vi "Configure Alarm Delay Math.vi"(0 "VISA resource name":refnum<visa-resource-name>, 5 "Math Channel (001)":string="001", 7 "Alarm Delay Time":cluster{"Hour":i32, "Min":i32, "Sec":i32}={"Hour"=0, "Min"=0, "Sec"=10} {"Sec" min=0 max=59; "Min" min=0 max=59; "Hour" min=0 max=24}, 11 "error in (no error)":errorcluster) -> (4 "VISA resource name out":refnum<visa-resource-name>, 6 "Math Channel":string, 15 "error out":errorcluster)   [LabVIEW 2020, in "Yokogawa GX Series.lvlib"]
doc: "Sets the alarm delay of a math channel.\n\nCommand: SAlmDlyMath"
uses:
  <instrlib>/Yokogawa GX Series/Yokogawa GX Series.lvlib
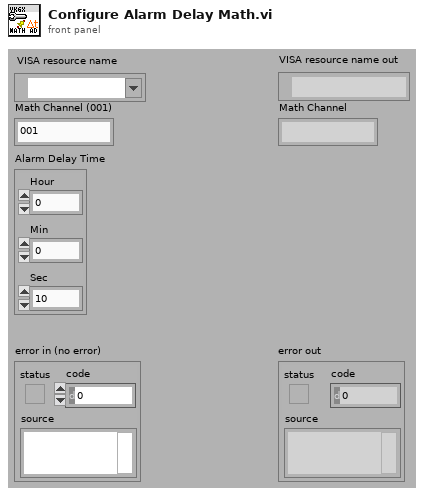
[diagram p1: front panel]
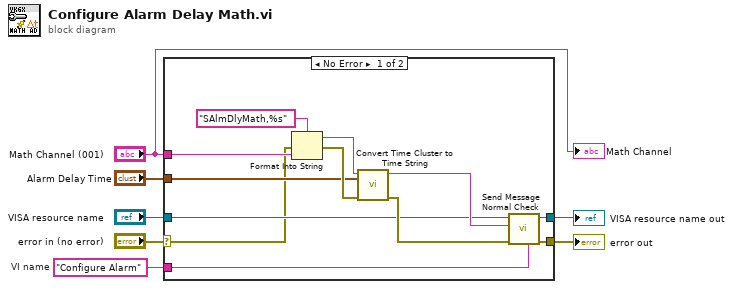
[diagram p0: block diagram]
diagram:
  w7 = "Configure Alarm"  # VI name
  n1 = case shown="No Error" "error in (no error)" {
    selector: "error in (no error)" -> [w8 w20]
    tunnel: w7 -> [w19 _]
    tunnel: [w18 w21] -> w6
    tunnel: [w17 w20] -> w5
    tunnel: "Alarm Delay Time" -> [w11 _]
    tunnel: "VISA resource name" -> [w10 w21]
    tunnel: "Math Channel (001)" -> [w9 _]
    frame No Error {
      n2 = Format Into String(format string="SAlmDlyMath,%s" ("形式文字列"), error in=w8, w9) -> (resulting string=w13:string, error out=w15:errorcluster)  [unwired: 1 in]
      n3 = call <instrlib>:"Convert Time Cluster to Time String.vi"("error in (no error)"=w15, "Time"=w11, "String"=w13) -> ("error out"=w14:errorcluster, "Time String"=w12:string)  [unwired: 7 in]
      n4 = call <instrlib>:"Send Message Normal Check.vi"("Source (\"\")"=w19, "error in (no error)"=w14, "Send Message (\"\")"=w12, "VISA resource name"=w10) -> ("error out"=w17:errorcluster, "VISA resource name out"=w18:refnum<visa-resource-name>)  [unwired: 2 in, 4 out]
    }
    frame Error {
    }
  }
  "error out" <- w5
  "VISA resource name out" <- w6
  "Math Channel" <- "Math Channel (001)"
